vi "Array to Vector3D.vi"(1 "Array":dbl[](array[numeric])) -> (0 "Vector3D":T1)   [LabVIEW 2013]
uses:
  controls/Vector3D Fingers.ctl
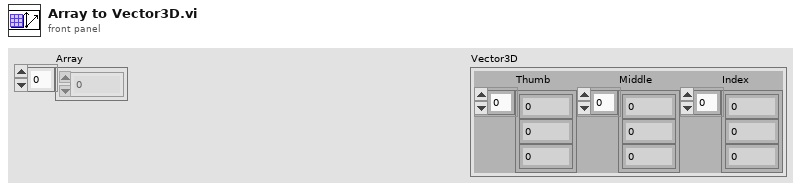
[diagram p1: front panel]
types:
  T1 = typedef "Vector3D Fingers.ctl" = cluster{"Thumb":dbl[], "Middle":dbl[], "Index":dbl[]}
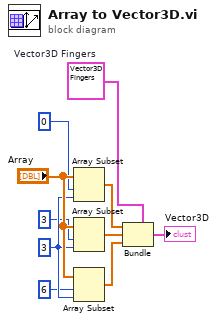
[diagram p0: block diagram]
diagram:
  w3 = 3 ("length")
  w10 = T1 {"Thumb"=[0.0, 0.0, 0.0], "Middle"=[0.0, 0.0, 0.0], "Index"=[0.0, 0.0, 0.0]}  # Vector3D Fingers
  n1 = Array Subset(array="Array", index=0, length=w3) -> (w7:dbl[])
  n2 = Array Subset(array="Array", index=3, length=w3) -> (w6:dbl[])
  n3 = Array Subset(array="Array", index=6, length=w3) -> (w5:dbl[])
  n4 = Bundle(cluster=w10, "Thumb"=w7, "Middle"=w6, "Index"=w5) -> (→"Vector3D":T1)
